vi "OE1022D_Configure Ref Phase Channel B.vi"(0 "VISA resource name":refnum<visa-resource-name>, 1 "Reference Source":u8(ring) items=["External", "Internal", "Internal Sweep", "Channel A"], 2 "External Ref Trigger":u8(ring)=1 items=["TTL Pos", "TTL Neg", "Sine Zero Crossing"], 3 "Internal Frequency(Hz)":sgl=1000.0 format="%.3f", 4 "Auto Phase (T: Enabled)":bool=TRUE, 5 "error in (no error)":errorcluster, 6 "Sweep Mode":u8(ring) items=["Linear", "Log"], 7 "Linear Step Frequency(Hz)":sgl=1000.0 format="%.3f", 8 "Start Frequency(Hz)":sgl=1000.0 format="%.3f", 9 "Log Step Percent(%)":sgl=10.0 format="%.3f", 10 "Stop Frequency(Hz)":sgl=5000.0 format="%.3f", 11 "Sweep Run Mode":u8(ring) items=["Stop", "Single", "Loop"], 12 "Step Time(ms)":sgl=1000.0 min=1 max=100000, 15 "Manual Phase  (degree)":sgl format="%.2f") -> (14 "VISA resource name out":refnum<visa-resource-name>, 19 "error out":errorcluster)   [LabVIEW 2022 SP3]
doc: "Configures the reference source and the internal oscillator."
panel:
  out "结果字符串":string
  # "Signal Generator"
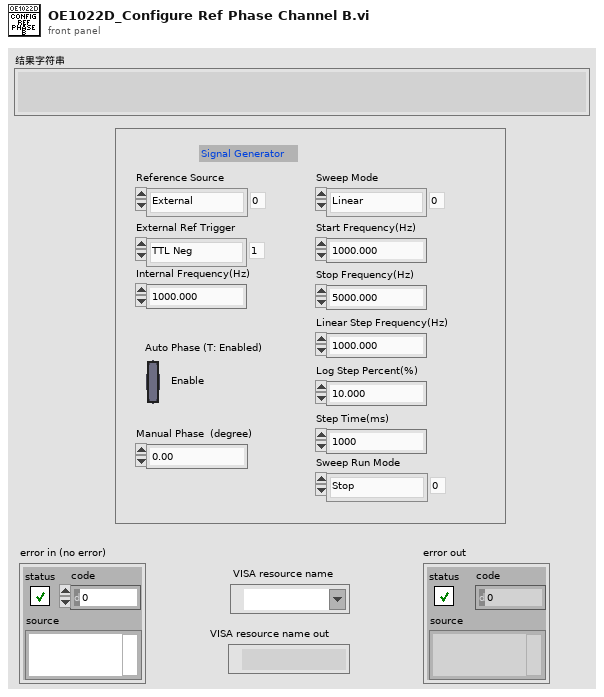
[diagram p1: front panel]
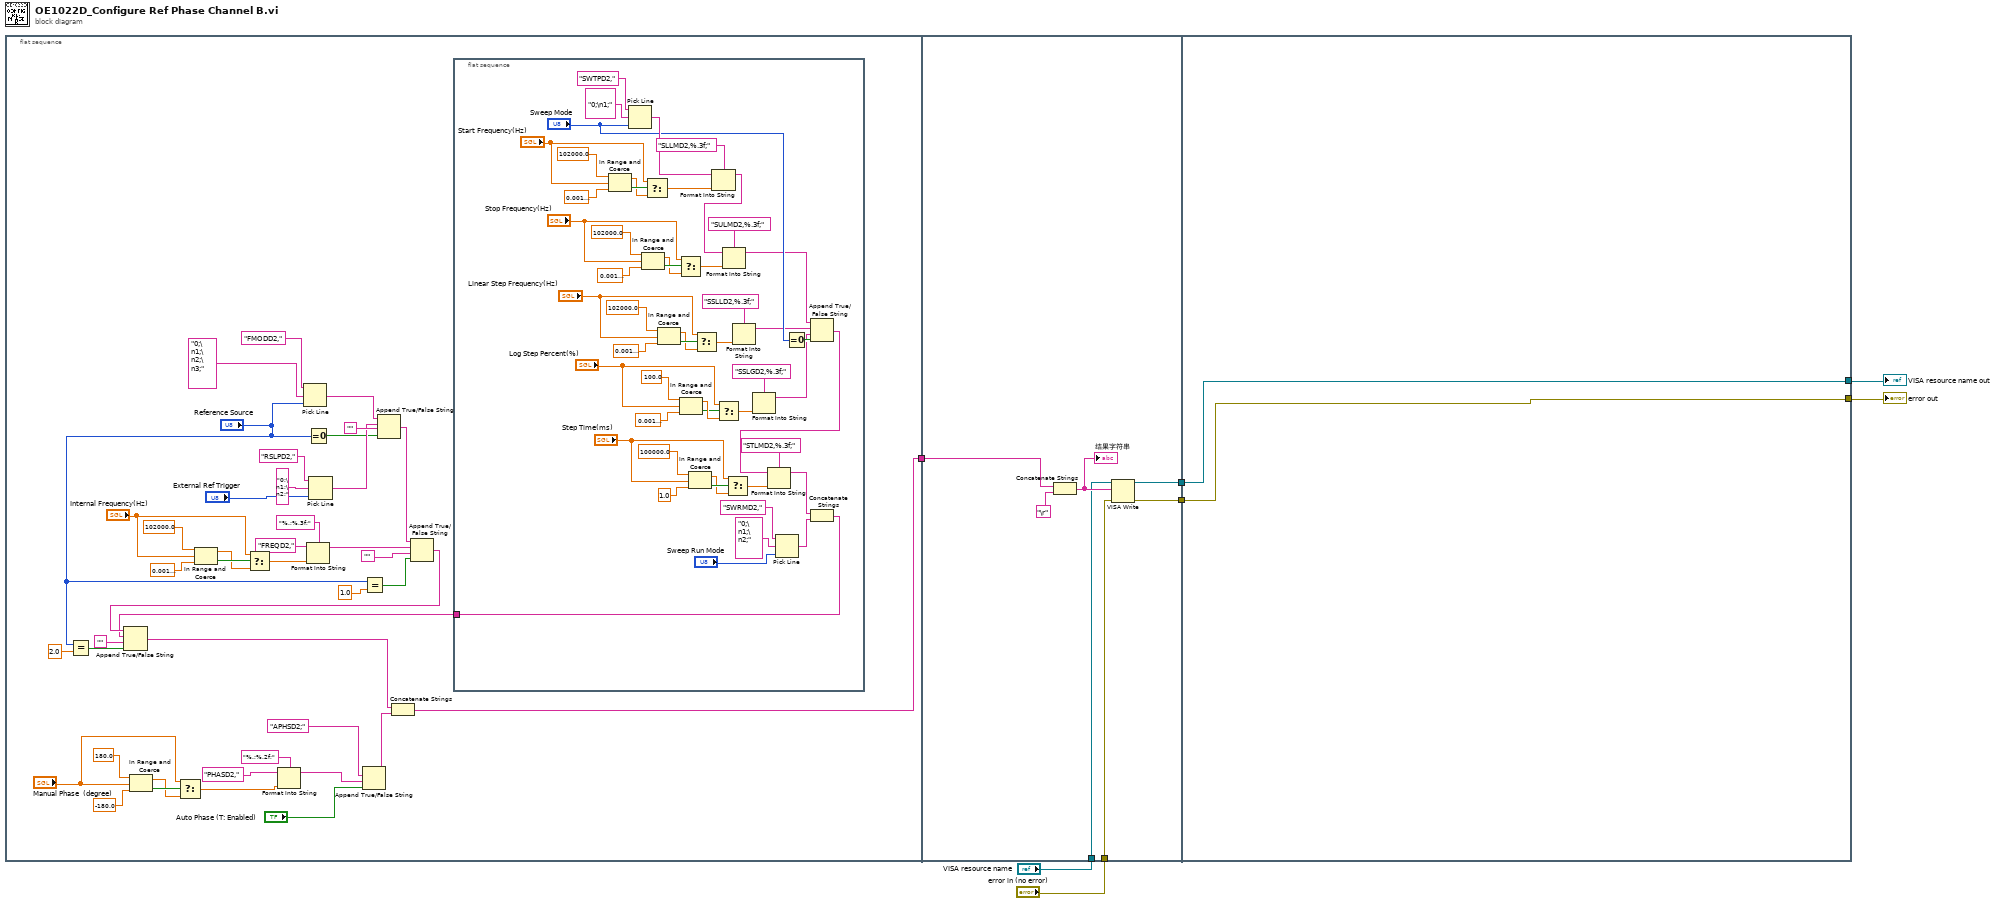
[diagram p0: block diagram]
diagram:
  n1 = flat-sequence {
    tunnel: [w22] -> w5
    tunnel: w5 -> [w105]
    tunnel: "VISA resource name" -> [w104]
    tunnel: "error in (no error)" -> [w103]
    tunnel: [w102] -> w4
    tunnel: [w101] -> w3
    tunnel: [w109] -> w7
    tunnel: [w108] -> w6
    tunnel: w4 -> [w109]
    tunnel: w3 -> [w108]
    frame #0 {
      n2 = Equal?(x="Reference Source", y=2.0) -> (x = y?=w30:bool)
      n3 = In Range and Coerce(upper limit=sgl 180.0 ("上限"), x="Manual Phase  (degree)", lower limit=sgl -180.0 ("下限")) -> (coerced(x)=w16:sgl, In Range?=w18:bool)
      n4 = Select(t="Manual Phase  (degree)", s=w18, f=w16) -> (s? t:f=w15:sgl)
      n5 = In Range and Coerce(upper limit=sgl 102000.0 ("上限"), x="Internal Frequency(Hz)", lower limit=sgl 0.001 ("下限")) -> (coerced(x)=w32:sgl, In Range?=w36:bool)
      n6 = Select(t="Internal Frequency(Hz)", s=w36, f=w32) -> (s? t:f=w48:sgl)
      n7 = Format Into String(format string="%.;%.2f;" ("格式字符串"), initial string="PHASD2,", w15) -> (resulting string=w19:string)  [unwired: 1 in, 1 out]
      n8 = Pick Line(string ("")="FMODD2,", multi-line string="0;\n1;\n2;\n3;", line index="Reference Source") -> (output string=w37:string)
      n9 = Format Into String(format string="%.;%.3f;", initial string="FREQD2,", w48) -> (resulting string=w26:string)  [unwired: 1 in, 1 out]
      n10 = Equal To 0?(x="Reference Source") -> (x = 0?=w38:bool)
      n11 = Pick Line(string ("")="RSLPD2,", multi-line string="0;\n1;\n2;", line index="External Ref Trigger") -> (output string=w40:string)
      n12 = Append True/False String(1:"Auto Phase (T: Enabled)", 2:w19, 3:"APHSD2;" ("string (\"\")")) -> (0:w9:string)  [unwired: 1 in]
      n13 = Equal?(x="Reference Source", y=1.0) -> (x = y?=w23:bool)
      n14 = Append True/False String(1:w38, 2:"" ("false string"), 3:w40, 4:w37) -> (0:w39:string)
      n15 = Append True/False String(1:w23, 2:"" ("false string"), 3:w26, 4:w39) -> (0:w29:string)
      n16 = Append True/False String(1:w30, 2:"", 3:w27, 4:w29) -> (0:w21:string)
      n17 = Concatenate Strings(w21, w9) -> (w22:string)
      n18 = flat-sequence {
        tunnel: [w56] -> w27
        frame #0 {
          n19 = In Range and Coerce(upper limit=sgl 102000.0 ("上限"), x="Start Frequency(Hz)", lower limit=sgl 0.001 ("下限")) -> (coerced(x)=w92:sgl, In Range?=w96:bool)
          n20 = Pick Line(string ("")="SWTPD2,", multi-line string="0;\n1;", line index="Sweep Mode") -> (output string=w60:string)
          n21 = In Range and Coerce(upper limit=sgl 102000.0 ("上限"), x="Stop Frequency(Hz)", lower limit=sgl 0.001 ("下限")) -> (coerced(x)=w86:sgl, In Range?=w89:bool)
          n22 = Select(t="Start Frequency(Hz)", s=w96, f=w92) -> (s? t:f=w98:sgl)
          n23 = In Range and Coerce(upper limit=sgl 102000.0 ("上限"), x="Linear Step Frequency(Hz)", lower limit=sgl 0.001 ("下限")) -> (coerced(x)=w79:sgl, In Range?=w82:bool)
          n24 = Select(t="Stop Frequency(Hz)", s=w89, f=w86) -> (s? t:f=w91:sgl)
          n25 = In Range and Coerce(upper limit=sgl 100.0 ("上限"), x="Log Step Percent(%)", lower limit=sgl 0.001 ("下限")) -> (coerced(x)=w77:sgl, In Range?=w74:bool)
          n26 = In Range and Coerce(upper limit=sgl 100000.0 ("上限"), x="Step Time(ms)", lower limit=sgl 1.0 ("下限")) -> (coerced(x)=w65:sgl, In Range?=w68:bool)
          n27 = Select(t="Linear Step Frequency(Hz)", s=w82, f=w79) -> (s? t:f=w84:sgl)
          n28 = Format Into String(format string="SLLMD2,%.3f;", initial string=w60, w98) -> (resulting string=w59:string)  [unwired: 1 in, 1 out]
          n29 = Select(t="Log Step Percent(%)", s=w74, f=w77) -> (s? t:f=w72:sgl)
          n30 = Format Into String(format string="SULMD2,%.3f;", initial string=w59, w91) -> (resulting string=w51:string)  [unwired: 1 in, 1 out]
          n31 = Select(t="Step Time(ms)", s=w68, f=w65) -> (s? t:f=w70:sgl)
          n32 = Format Into String(format string="SSLLD2,%.3f;", w84) -> (resulting string=w53:string)  [unwired: 2 in, 1 out]
          n33 = Format Into String(format string="SSLGD2,%.3f;", w72) -> (resulting string=w52:string)  [unwired: 2 in, 1 out]
          n34 = Pick Line(string ("")="SWRMD2,", multi-line string="0;\n1;\n2;", line index="Sweep Run Mode") -> (output string=w58:string)
          n35 = Equal To 0?(x="Sweep Mode") -> (x = 0?=w55:bool)
          n36 = Append True/False String(1:w55, 2:w52, 3:w53, 4:w51) -> (0:w50:string)
          n37 = Format Into String(format string="STLMD2,%.3f;", initial string=w50, w70) -> (resulting string=w57:string)  [unwired: 1 in, 1 out]
          n38 = Concatenate Strings(w57, w58) -> (w56:string)
        }
      }
    }
    frame #1 {
      n39 = Concatenate Strings(w105, "\r") -> (w106:string)
      "结果字符串" <- w106
      n40 = VISA Write(VISA resource name=w104, write buffer=w106, error in (no error)=w103) -> (VISA resource name out=w102:refnum<visa-resource-name>, error out=w101:errorcluster)  [unwired: 1 out]
    }
    frame #2 {
    }
  }
  "error out" <- w6
  "VISA resource name out" <- w7
